vi "GPIO_Output (SubVI).vi"(8 "error in (no error)":errorcluster, 9 "GPIO Value":bool[](array[boolean]), 11 "VISA resource name":refnum<visa-resource-name>) -> (0 "error out":errorcluster, 3 "VISA resource name out":refnum<visa-resource-name>)   [LabVIEW 2018]
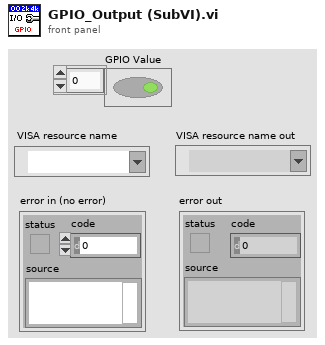
[diagram p1: front panel]
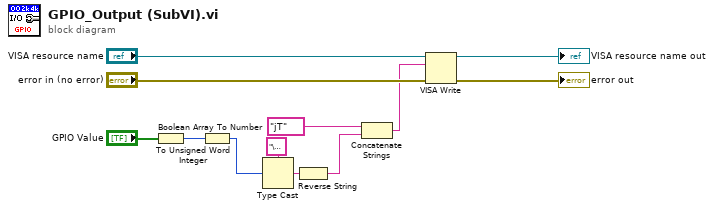
[diagram p0: block diagram]
diagram:
  n1 = Boolean Array To Number(Boolean array="GPIO Value") -> (number=w4:u32)
  n2 = To Unsigned Word Integer(number=w4) -> (unsigned 16bit integer=w3:u16)
  n3 = Type Cast(type="\u0000", x=w3) -> (*(type *) &x=w9:string)
  n4 = Reverse String(1:w9) -> (0:w10:string)
  n5 = Concatenate Strings("jT" ("string"), w10) -> (w6:string)
  n6 = VISA Write(VISA resource name="VISA resource name", write buffer=w6, error in (no error)="error in (no error)") -> (VISA resource name out=→"VISA resource name out":refnum<visa-resource-name>, error out=→"error out":errorcluster)  [unwired: 1 out]
